vi "oax_Call Tachless VI.vi"(8 "error in (no error)":errorcluster, 11 "scaled signal [EU]":waveform(dbl)={"t0"=timestamp(0 s since 1904-01-01), "dt"=0.0, "Y"=[]}) -> (0 "error out":errorcluster, 1 "orders list":dbl[](array[numeric]), 2 "speed profile":T1 {"speed [RPM]" format="%.2f"; "time [s]" format="%.2f"}, 3 "dup scaled signal [EU]":waveform(dbl))   [LabVIEW 2017]
uses:
  <vilib>/addons/Sound and Vibration/Order Analysis/Tach Process/SubVIs/speed profile.ctl
  <vilib>/addons/Sound and Vibration/Order Analysis/Tach Process/SoundVib_TachProcess.lvlib
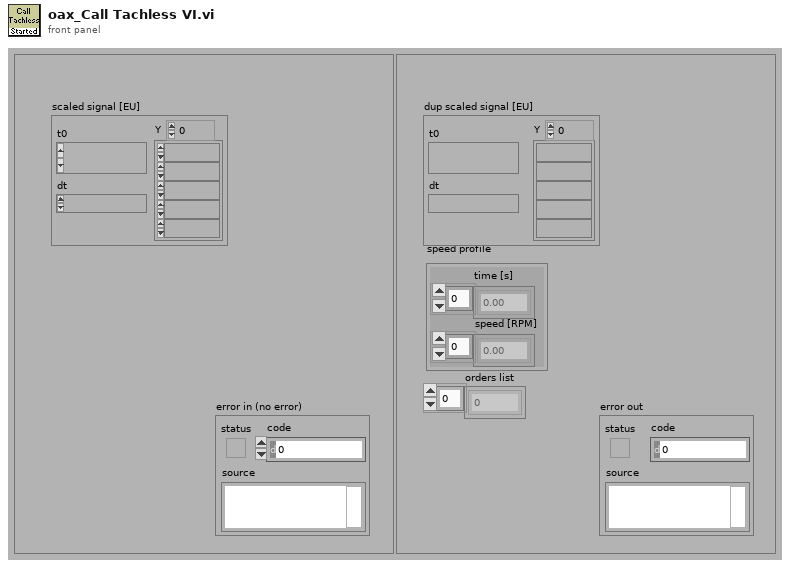
[diagram p1: front panel]
types:
  T1 = typedef "SoundVib_TachProcess.lvlib/speed profile.ctl" = cluster{"time [s]":dbl[], "speed [RPM]":dbl[]}
  T2 = typedef "speed profile.ctl" = cluster{"time [s]":dbl[], "speed [RPM]":dbl[]}
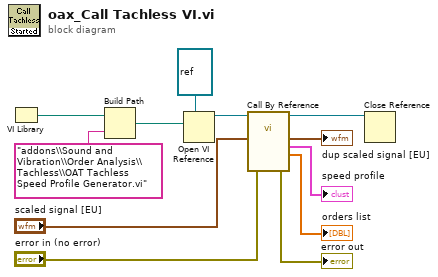
[diagram p0: block diagram]
diagram:
  n1 = VI Library() -> (path=w12:path)
  n2 = Build Path(base path=w12, name or relative path="addons\\Sound and Vibration\\Order Analysis\\Tachless\\OAT Tachless Speed Profile Generator.vi") -> (appended path=w10:path)
  n3 = Open VI Reference(type specifier VI Refnum (for type only)=refnum<vi> refnum, vi path=w10) -> (vi reference=w9:refnum<vi>)  [unwired: 4 in, 1 out]
  n4 = call-by-ref "?"(reference=w9, "error in (no error)"="error in (no error)", "scaled signal [EU]"="scaled signal [EU]") -> (reference out=w3:refnum<vi>, "error out"=→"error out":errorcluster, "orders list"=→"orders list":dbl[], "speed profile"=→"speed profile":T2, "dup scaled signal [EU]"=→"dup scaled signal [EU]":waveform(dbl))  [unwired: 5 in, 3 out]
  n5 = Close Reference(reference=w3) -> ()  [unwired: 1 in, 1 out]
